vi "SE FP Find red target.vi"(0 "Image In":T2, 1 "error in (no error)":errorcluster) -> (2 "Image Dst Out":T2, 3 "Nb Circles (Circle Detection 1)":i32, 4 "Camera Data":T1(array[cluster]), 5 "error out":errorcluster)   [LabVIEW 2014]
doc: "This VI takes in an image and finds a round, red target. It produces the target location and size."
uses:
  <vilib>/vision/Image Controls.llb/IMAQ Image.ctl
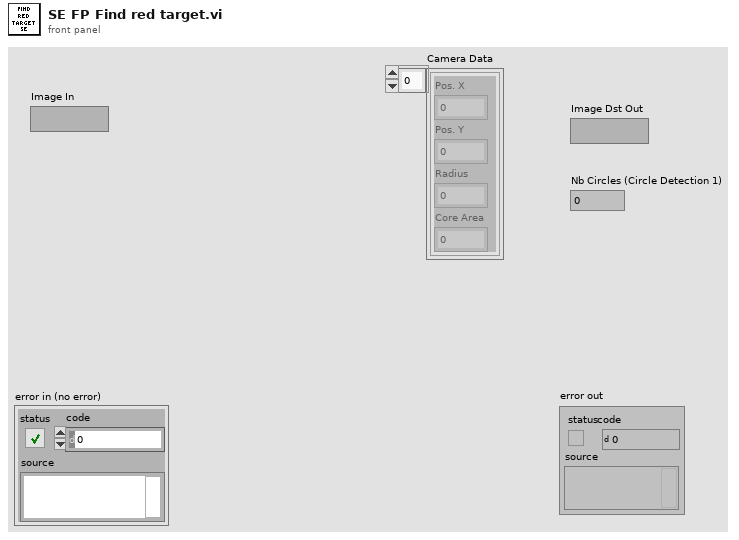
[diagram p1: front panel]
types:
  T1 = cluster{"Pos. X":i32, "Pos. Y":i32, "Radius":i32, "Core Area":i32}[]
  T2 = typedef "IMAQ Image.ctl" = refnum<image>
  T3 = cluster{"Pos. X":i32, "Pos. Y":i32, "Radius":i32, "Core Area":i32}
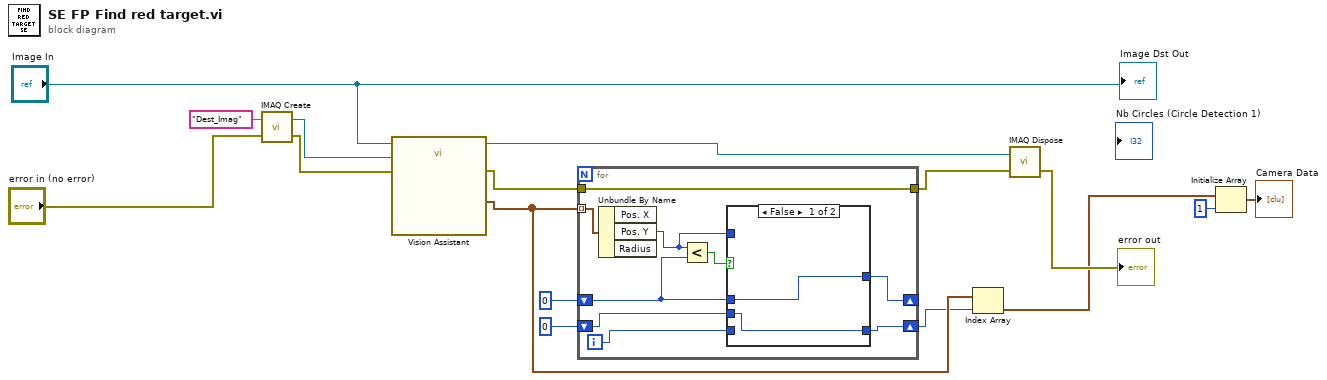
[diagram p0: block diagram]
diagram:
  n1 = call "IMAQ Create"("Image Name"="Dest_Imag", "error in (no error)"="error in (no error)") -> ("New Image"=w13:T2, "error out"=w14:errorcluster)  [unwired: 3 in]
  n2 = call "Vision Assistant"("Image In"="Image In", "Image Dst"=w13, "error in"=w14) -> ("Image Out"=w12:T2, "Circles Data (Circle Detection 1)"=w5:T1, "error out"=w9:errorcluster)  [unwired: 21 in, 1 out]
  n3 = for {
    tunnel: w9 -> [w25]
    tunnel: [w25] -> w8
    tunnel: w5 -> [w24] mode=indexing
    shift-right: [w21] -> _
    shift-left: 0 -> [w20]
    shift-right: [w17] -> w4
    shift-left: 0 -> [w19]
    i -> [w18]
    n4 = Unbundle By Name(w24) -> ("Pos. Y"=w22:i32)  [unwired: 2 out]
    n5 = Less?(x=w22, y=w20) -> (x < y?=w23:bool)
    n6 = case shown="False" w23 {
      tunnel: w22 -> [_ w29]
      tunnel: [w27 w29] -> w21
      tunnel: w20 -> [w27 _]
      tunnel: w19 -> [w26 _]
      tunnel: w18 -> [_ w28]
      tunnel: [w26 w28] -> w17
      frame False {
      }
      frame True {
      }
    }
  }
  n7 = Index Array(array=w5, index=w4) -> (element=w2:T3)
  n8 = call "IMAQ Dispose"("Image"=w12, "error in (no error)"=w8) -> ("error out"=→"error out":errorcluster)  [unwired: 1 in, 3 out]
  n9 = Initialize Array(w2, 1 ("dimension size")) -> (→"Camera Data":T1)
  "Image Dst Out" <- "Image In"
